vi "LeCroy Wave Series Sequence Acquisition.vi"() -> ()   [LabVIEW 2015]
doc: "This example shows how to use autosetup and acquire a sequence waveform on a single channel. Sequence waveform consists of a number of segments. Each segment is acquired when triggering condition is met."
uses:
  <instrlib>/LeCroy Wave Series/Public/Data/Read Single Sequence.vi
  <instrlib>/LeCroy Wave Series/LeCroy Wave Series.lvlib
panel:
  in  "Number of Segments (2)":u16=2
  in  "Source (0: Channel 1)":u16(ring) items=["Channel 1", "Channel 2", "Channel 3", "Channel 4", "Memory 1", "Memory 2", "Memory 3", "Memory 4", "Function 1", "Function 2", "Function 3", "Function 4", "Function 5", "Function 6", "Function 7", "Function 8"]
  out "Waveform Data":waveform(dbl)(graph)
  in  "Timeout (10000 ms)":u32=10000
  in  "VISA resource name":refnum<visa-resource-name>
  # "(c) 2008 - 2012 NATIONAL INSTRUMENTS.  ALL RIGHTS RESERVED."
  # "Directions:\n\n1. Setup the scope to be able to successfully single trigger on a signal applied to the channel selected in the \"Source\" control using \"RealTime\" mode/\n\n2. On this front panel, enter the VISA Resource name for your scope. (e.g. VICP::123.45.67.8 for TCP/IP, GPIB::5::INSTR for GPIB). Modify the timeout if necessary.\n\n3. Enter  the number of segments to acquire.\n\n4. Run the VI to trigger the scope an to readback the data."
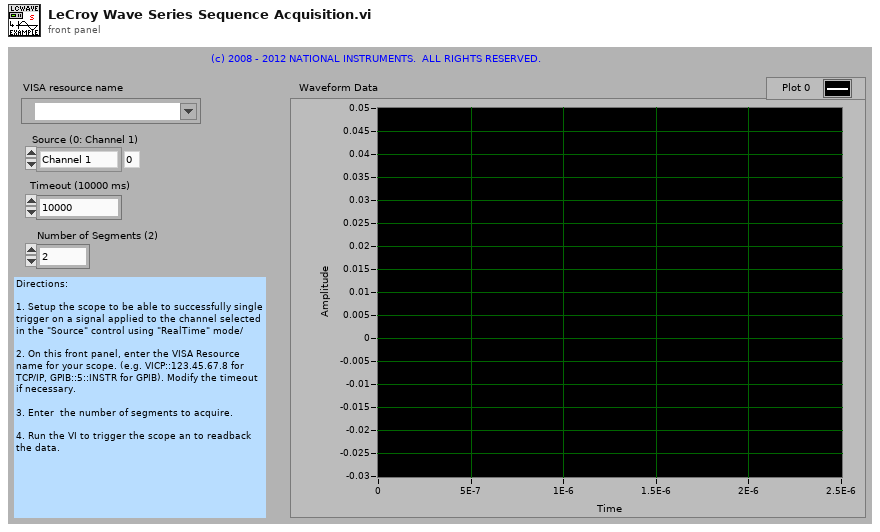
[diagram p1: front panel]
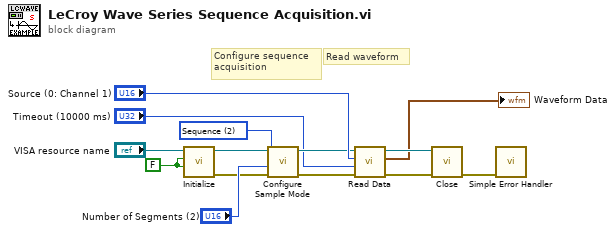
[diagram p0: block diagram]
diagram:
  w3 = FALSE ("ID Query? (T: Yes)")
  w5 = u16 2 items=["RealTime", "RIS", "Sequence", "Roll", "WaveStream"] ("Sample Mode (0: RealTime)")
  # "Read waveform"
  # "Configure sequence\nacquisition"
  n1 = call <instrlib>:"Initialize.vi"("Reset? (T: Yes)"=w3, "ID Query? (T: Yes)"=w3, "VISA resource name"="VISA resource name") -> ("error out"=w2:errorcluster, "VISA resource name out"=w1:refnum<visa-resource-name>)  [unwired: 7 in]
  n2 = call <instrlib>:"Configure Sample Mode.vi"("error in (no error)"=w2, "Number of Segments (2)"="Number of Segments (2)", "Sample Mode (0: RealTime)"=w5, "VISA resource name"=w1) -> ("error out"=w7:errorcluster, "VISA resource name out"=w8:refnum<visa-resource-name>)  [unwired: 6 in]
  n3 = call-poly <instrlib>:"Read Data.vi"("error in (no error)"=w7, "Timeout (10000 ms)"="Timeout (10000 ms)", "Source (0: Channel 1)"="Source (0: Channel 1)", "VISA resource name"=w8) -> ("error out"=w12:errorcluster, "Waveform Data"=→"Waveform Data":waveform(dbl), "VISA resource name out"=w13:refnum<visa-resource-name>)  [unwired: 5 in]
  n4 = call <instrlib>:"Close.vi"("error in (no error)"=w12, "VISA resource name"=w13) -> ("error out"=w14:errorcluster)  [unwired: 9 in]
  n5 = call <vilib>:"Simple Error Handler.vi"("error in (no error)"=w14) -> ()  [unwired: 4 in, 5 out]
